vi "Begin.vi"() -> (0 "error out":errorcluster)   [LabVIEW 2013]
doc: "Called before other user functions, this VI is expected to open initial I/O refnums, load in file data, and do all program initialization. Notice that the <B>error out</B> terminal is simply used for data flow. Wiring it to other structures or subVIs ensures that this VI runs first."
uses:
  <vilib>/Rock Robotics/WPI/DriverStation/WPI_DriverStationRobotMode2.ctl
  <vilib>/Rock Robotics/WPI/Joystick/WPI_JoystickDeviceEnum.ctl
  <vilib>/Rock Robotics/SystemInterfaces/DIO/FPGA_DIOPWMChannel.ctl
  <vilib>/Rock Robotics/SystemInterfaces/DIO/FPGA_DIOChannel.ctl
  <vilib>/Rock Robotics/SystemInterfaces/AI/FPGA_AIChannel.ctl
  <vilib>/Rock Robotics/SystemInterfaces/Typedef/FPGA_TypedefAnalogModule.ctl
  <vilib>/Rock Robotics/SystemInterfaces/DIO/FPGA_DIORelayChannel.ctl
  <vilib>/Rock Robotics/SystemInterfaces/Typedef/FPGA_TypedefDigitalModule.ctl
  Robot Global Data.vi
  <vilib>/Rock Robotics/WPI/MotorControl/WPI_MotorControlOpen Talon.vi
panel:
  out "error out 3":errorcluster
  out "error out 2":errorcluster
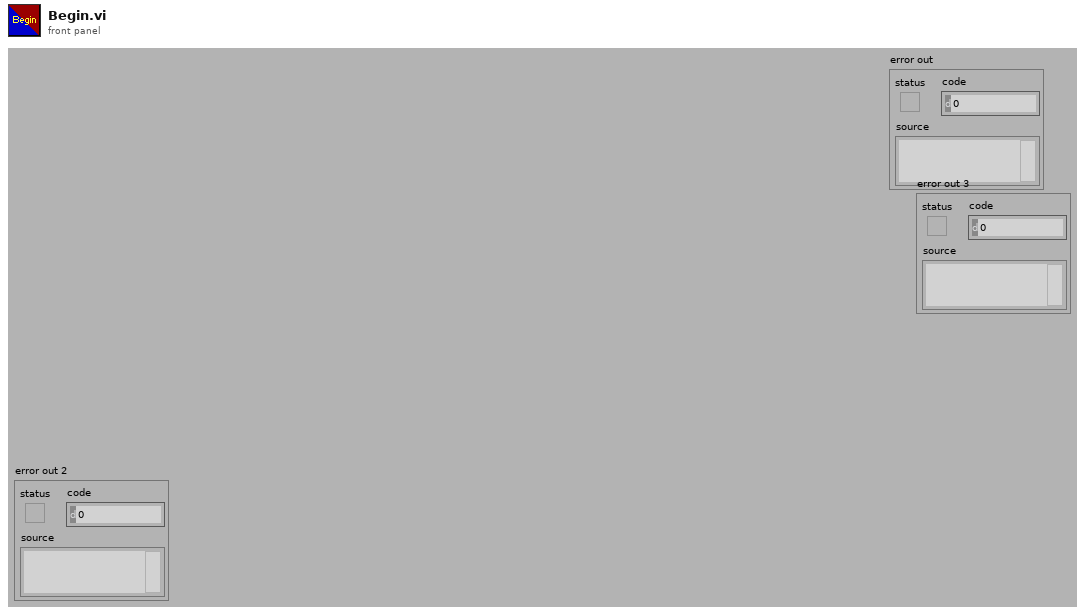
[diagram p1: front panel]
types:
  T1 = typedef "FPGA_DIOChannel.ctl" = enum8{"DIO 1", "DIO 2", "DIO 3", "DIO 4", "DIO 5", "DIO 6", "DIO 7", "DIO 8", "DIO 9", "DIO 10", "DIO 11", "DIO 12", "DIO 13", "DIO 14", "Invalid"}
  T2 = typedef "FPGA_TypedefDigitalModule.ctl" = enum16{"Digital Module 1", "Digital Module 2"}
  T3 = typedef "FPGA_DIORelayChannel.ctl" = enum8{"Relay 1", "Relay 2", "Relay 3", "Relay 4", "Relay 5", "Relay 6", "Relay 7", "Relay 8", "Invalid"}
  T4 = typedef "FPGA_DIOPWMChannel.ctl" = enum8{"PWM 1", "PWM 2", "PWM 3", "PWM 4", "PWM 5", "PWM 6", "PWM 7", "PWM 8", "PWM 9", "PWM 10", "Invalid"}
  T5 = typedef "FPGA_TypedefAnalogModule.ctl" = enum16{"Analog Module 1", "Analog Module 2"}
  T6 = typedef "FPGA_AIChannel.ctl" = enum8{"AI 1", "AI 2", "AI 3", "AI 4", "AI 5", "AI 6", "AI 7", "AI 8", "Invalid"}
  T7 = typedef "WPI_JoystickDeviceEnum.ctl" = enum16{"USB 1", "USB 2", "USB 3", "USB 4", "Kinect 1", "Kinect 2"}
  T8 = typedef "WPI_DriverStationRobotMode2.ctl" = enum16{"Autonomous Disabled", "Autonomous Enabled", "Teleop Disabled", "Teleop Enabled", "Timeout", "Finish", "Test Disabled", "Test Enabled"}
  T9 = typedef "WPI_JoystickDevRef.ctl" = cluster{"Device":T7}
  T10 = typedef "WPI_MotorControlDeviceRef.ctl" = cluster{"DeviceStatus":errorcluster, "Type":enum16{"PWM", "CAN"}, "PWM":cluster{"Digital Module":T2, "PWM Channel":T4, "DeadBand":T11}, "CAN":cluster{"Device Number":u8, "Control Mode":T12, "Semaphore":T13, "Max Vout":dbl}, "Invert":bool, "TransformRef":T14, "InvTransformRef":T14}
  T11 = typedef "WPI_PWMDeadband.ctl" = cluster{"Name":string, "maxPositivePwm":i32, "minPositivePwm":i32, "centerPwm":i32, "maxNegativePwm":i32, "minNegativePwm":i32, "angularRange":u16}
  T12 = typedef "WPI_CANJaguar_ControlMode.ctl" = enum8{"Percent VBus", "Current", "Speed", "Position", "Voltage"}
  T13 = typedef "Semaphore RefNum" = refnum<k1>
  T14 = typedef "WPI_PWMTransform_ConPane.ctl" = refnum<vi>
  T15 = typedef "WPI_RelayDevRef.ctl" = cluster{"DevStatus":errorcluster, "Relay Channel":T3, "Digital Module":T2, "Relay Direction":T16}
  T16 = typedef "WPI_RelayDirection.ctl" = enum16{"Both directions", "Forward only", "Reverse only"}
  T17 = typedef "WPI_DigitalInputDevRef.ctl" = cluster{"DevStatus":errorcluster, "DIO Channel":T1, "Digital Module":T2}
  T18 = typedef "WPI_AnalogChannelDevRef.ctl" = cluster{"DevStatus":errorcluster, "Analog Module":T5, "Analog Channel":T6}
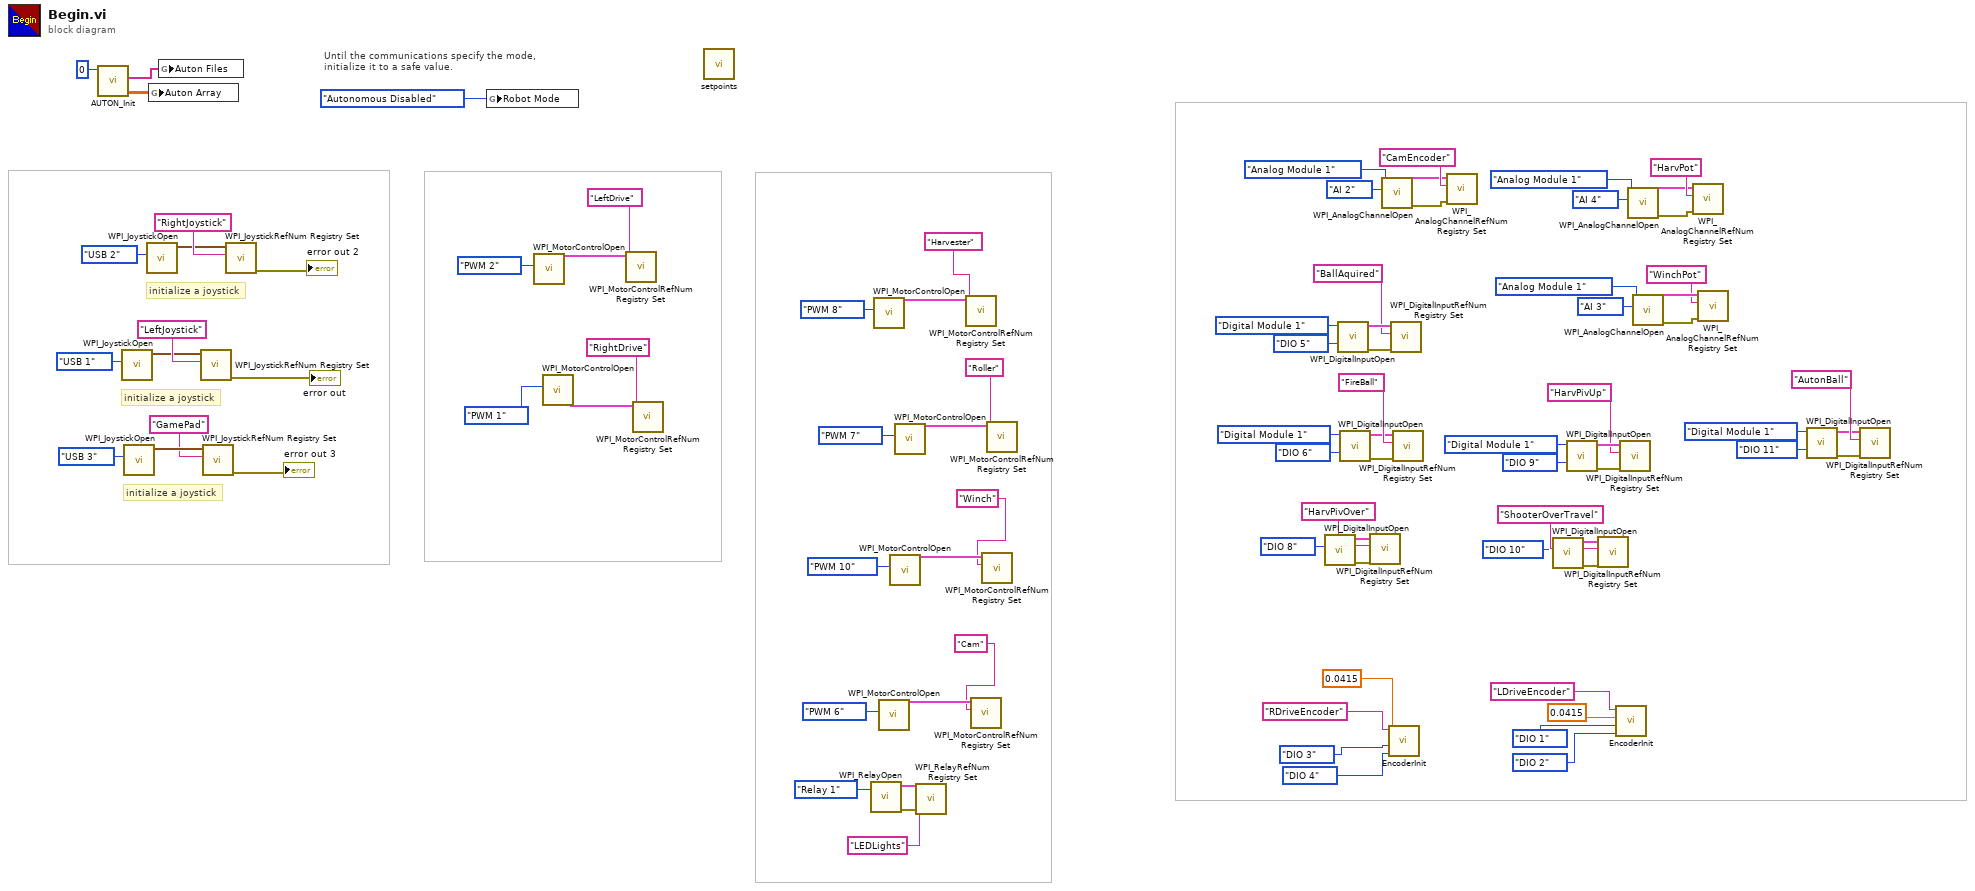
[diagram p0: block diagram]
diagram:
  # "initialize a joystick"
  # "initialize a joystick"
  # "initialize a joystick"
  # "Until the communications specify the mode,\ninitialize it to a safe value."
  n1 = call "AUTON_Init.vi"("Default File"=0) -> ("Auton Array"=w11:dbl[][], "Auton Files"=w10:string[])  [unwired: 8 in, 1 out]
  n2 = call <vilib>:"WPI_JoystickOpen.vi"("JoystickDevice"=WPI_JoystickDeviceEnum."USB 1") -> ("JoystickDevRef"=w87:T9)  [unwired: 10 in]
  n3 = call <vilib>:"WPI_JoystickOpen.vi"("JoystickDevice"=WPI_JoystickDeviceEnum."USB 3") -> ("JoystickDevRef"=w62:T9)  [unwired: 10 in]
  n4 = call <vilib>:"WPI_JoystickOpen.vi"("JoystickDevice"=WPI_JoystickDeviceEnum."USB 2") -> ("JoystickDevRef"=w83:T9)  [unwired: 10 in]
  n5 = global write "Robot Global Data.vi" "Auton Array"(w11) -> ()
  n6 = global write "Robot Global Data.vi" "Auton Files"(w10) -> ()
  n7 = call <vilib>:"WPI_JoystickRefNum Registry Set.vi"("refnum name"="LeftJoystick", "JoystickDevRef"=w87) -> ("error out"=→"error out":errorcluster)  [unwired: 8 in, 1 out]
  n8 = call <vilib>:"WPI_JoystickRefNum Registry Set.vi"("refnum name"="GamePad", "JoystickDevRef"=w62) -> ("error out"=→"error out 3":errorcluster)  [unwired: 8 in, 1 out]
  n9 = call <vilib>:"WPI_JoystickRefNum Registry Set.vi"("refnum name"="RightJoystick", "JoystickDevRef"=w83) -> ("error out"=→"error out 2":errorcluster)  [unwired: 8 in, 1 out]
  n10 = global write "Robot Global Data.vi" "Robot Mode"(WPI_DriverStationRobotMode2."Autonomous Disabled" ("Robot Mode")) -> ()
  n11 = call-poly <vilib>:"WPI_MotorControlOpen.vi"("PWM Channel"=FPGA_DIOPWMChannel."PWM 2") -> ("MotorControlDeviceRef"=w79:T10)  [unwired: 9 in, 1 out]
  n12 = call-poly <vilib>:"WPI_MotorControlOpen.vi"("PWM Channel"=FPGA_DIOPWMChannel."PWM 1") -> ("MotorControlDeviceRef"=w76:T10)  [unwired: 9 in, 1 out]
  n13 = call <vilib>:"WPI_MotorControlRefNum Registry Set.vi"("refnum name"="LeftDrive", "MotorControlDevRef"=w79) -> ()  [unwired: 8 in, 2 out]
  n14 = call <vilib>:"WPI_MotorControlRefNum Registry Set.vi"("refnum name"="RightDrive", "MotorControlDevRef"=w76) -> ()  [unwired: 8 in, 2 out]
  n15 = call "setpoints.vi"() -> ()  [unwired: 12 in]
  n16 = call <vilib>:"WPI_RelayOpen.vi"("Relay Channel"=FPGA_DIORelayChannel."Relay 1") -> ("error out"=w8:errorcluster, "RelayDevRef"=w7:T15)  [unwired: 9 in]
  n17 = call-poly <vilib>:"WPI_MotorControlOpen.vi"("PWM Channel"=FPGA_DIOPWMChannel."PWM 8") -> ("MotorControlDeviceRef"=w73:T10)  [unwired: 9 in, 1 out]
  n18 = call-poly <vilib>:"WPI_MotorControlOpen.vi"("PWM Channel"=FPGA_DIOPWMChannel."PWM 6") -> ("MotorControlDeviceRef"=w44:T10)  [unwired: 9 in, 1 out]
  n19 = call-poly <vilib>:"WPI_MotorControlOpen.vi"("PWM Channel"=FPGA_DIOPWMChannel."PWM 10") -> ("MotorControlDeviceRef"=w46:T10)  [unwired: 9 in, 1 out]
  n20 = call-poly <vilib>:"WPI_MotorControlOpen.vi"("PWM Channel"=FPGA_DIOPWMChannel."PWM 7") -> ("MotorControlDeviceRef"=w71:T10)  [unwired: 9 in, 1 out]
  n21 = call <vilib>:"WPI_RelayRefNum Registry Set.vi"("error in (no error)"=w8, "refnum name"="LEDLights", "RelayDevRef"=w7) -> ()  [unwired: 7 in, 2 out]
  n22 = call <vilib>:"WPI_MotorControlRefNum Registry Set.vi"("refnum name"="Harvester", "MotorControlDevRef"=w73) -> ()  [unwired: 8 in, 2 out]
  n23 = call <vilib>:"WPI_MotorControlRefNum Registry Set.vi"("refnum name"="Cam", "MotorControlDevRef"=w44) -> ()  [unwired: 8 in, 2 out]
  n24 = call <vilib>:"WPI_MotorControlRefNum Registry Set.vi"("refnum name"="Winch", "MotorControlDevRef"=w46) -> ()  [unwired: 8 in, 2 out]
  n25 = call <vilib>:"WPI_MotorControlRefNum Registry Set.vi"("refnum name"="Roller", "MotorControlDevRef"=w71) -> ()  [unwired: 8 in, 2 out]
  n26 = call <vilib>:"WPI_DigitalInputOpen.vi"("DIO Channel"=FPGA_DIOChannel."DIO 8") -> ("error out"=w48:errorcluster, "DigitalInputDevRef"=w49:T17)  [unwired: 9 in]
  n27 = call <vilib>:"WPI_DigitalInputOpen.vi"("DIO Channel"=FPGA_DIOChannel."DIO 5", "Digital Module (Module 1)"=FPGA_TypedefDigitalModule."Digital Module 1") -> ("error out"=w69:errorcluster, "DigitalInputDevRef"=w68:T17)  [unwired: 8 in]
  n28 = call <vilib>:"WPI_DigitalInputOpen.vi"("DIO Channel"=FPGA_DIOChannel."DIO 6", "Digital Module (Module 1)"=FPGA_TypedefDigitalModule."Digital Module 1") -> ("error out"=w32:errorcluster, "DigitalInputDevRef"=w33:T17)  [unwired: 8 in]
  n29 = call <vilib>:"WPI_DigitalInputRefNum Registry Set.vi"("error in (no error)"=w48, "refnum name"="HarvPivOver", "DigitalInputDevRef"=w49) -> ()  [unwired: 7 in, 2 out]
  n30 = call <vilib>:"WPI_AnalogChannelOpen.vi"("Analog Channel"=FPGA_AIChannel."AI 2", "Analog Module (Module 1)"=FPGA_TypedefAnalogModule."Analog Module 1") -> ("error out"=w38:errorcluster, "AIDeviceRef"=w37:T18)  [unwired: 8 in]
  n31 = call "EncoderInit.vi"("refnum name"="RDriveEncoder", "DistancePerCount"=0.0415, "DIO Channel"=FPGA_DIOChannel."DIO 3", "DIO Channel 2"=FPGA_DIOChannel."DIO 4") -> ()  [unwired: 7 in]
  n32 = call <vilib>:"WPI_DigitalInputRefNum Registry Set.vi"("error in (no error)"=w69, "refnum name"="BallAquired", "DigitalInputDevRef"=w68) -> ()  [unwired: 7 in, 2 out]
  n33 = call <vilib>:"WPI_DigitalInputRefNum Registry Set.vi"("error in (no error)"=w32, "refnum name"="FireBall", "DigitalInputDevRef"=w33) -> ()  [unwired: 7 in, 2 out]
  n34 = call <vilib>:"WPI_AnalogChannelRefNum Registry Set.vi"("error in (no error)"=w38, "refnum name"="CamEncoder", "AIDeviceRef"=w37) -> ()  [unwired: 7 in, 2 out]
  n35 = call <vilib>:"WPI_DigitalInputOpen.vi"("DIO Channel"=FPGA_DIOChannel."DIO 10") -> ("error out"=w16:errorcluster, "DigitalInputDevRef"=w15:T17)  [unwired: 9 in]
  n36 = call <vilib>:"WPI_DigitalInputOpen.vi"("DIO Channel"=FPGA_DIOChannel."DIO 9", "Digital Module (Module 1)"=FPGA_TypedefDigitalModule."Digital Module 1") -> ("error out"=w21:errorcluster, "DigitalInputDevRef"=w20:T17)  [unwired: 8 in]
  n37 = call <vilib>:"WPI_DigitalInputRefNum Registry Set.vi"("error in (no error)"=w16, "refnum name"="ShooterOverTravel", "DigitalInputDevRef"=w15) -> ()  [unwired: 7 in, 2 out]
  n38 = call "EncoderInit.vi"("refnum name"="LDriveEncoder", "DistancePerCount"=0.0415, "DIO Channel"=FPGA_DIOChannel."DIO 1", "DIO Channel 2"=FPGA_DIOChannel."DIO 2") -> ()  [unwired: 7 in]
  n39 = call <vilib>:"WPI_DigitalInputRefNum Registry Set.vi"("error in (no error)"=w21, "refnum name"="HarvPivUp", "DigitalInputDevRef"=w20) -> ()  [unwired: 7 in, 2 out]
  n40 = call <vilib>:"WPI_AnalogChannelOpen.vi"("Analog Channel"=FPGA_AIChannel."AI 4", "Analog Module (Module 1)"=FPGA_TypedefAnalogModule."Analog Module 1") -> ("error out"=w28:errorcluster, "AIDeviceRef"=w27:T18)  [unwired: 8 in]
  n41 = call <vilib>:"WPI_AnalogChannelOpen.vi"("Analog Channel"=FPGA_AIChannel."AI 3", "Analog Module (Module 1)"=FPGA_TypedefAnalogModule."Analog Module 1") -> ("error out"=w59:errorcluster, "AIDeviceRef"=w60:T18)  [unwired: 8 in]
  n42 = call <vilib>:"WPI_AnalogChannelRefNum Registry Set.vi"("error in (no error)"=w28, "refnum name"="HarvPot", "AIDeviceRef"=w27) -> ()  [unwired: 7 in, 2 out]
  n43 = call <vilib>:"WPI_AnalogChannelRefNum Registry Set.vi"("error in (no error)"=w59, "refnum name"="WinchPot", "AIDeviceRef"=w60) -> ()  [unwired: 7 in, 2 out]
  n44 = call <vilib>:"WPI_DigitalInputOpen.vi"("DIO Channel"=FPGA_DIOChannel."DIO 11", "Digital Module (Module 1)"=FPGA_TypedefDigitalModule."Digital Module 1") -> ("error out"=w1:errorcluster, "DigitalInputDevRef"=w2:T17)  [unwired: 8 in]
  n45 = call <vilib>:"WPI_DigitalInputRefNum Registry Set.vi"("error in (no error)"=w1, "refnum name"="AutonBall", "DigitalInputDevRef"=w2) -> ()  [unwired: 7 in, 2 out]
